vi "Frequency Changer.vi"() -> ()   [LabVIEW 2025]
uses:
  Globals/Speaker VISA Global.vi
  Globals/Motor VISA Global.vi
  Globals/Wire VISA Global.vi
  Globals/Light VISA Global.vi
  Globals/Solenoid VISA Global.vi
  Globals/Touch VISA Global.vi
panel:
  out "Success?":bool
  in  "Cancel Button":bool
  in  "OK Button":bool
  in  "Frequency":i16
  in  "Module":string(combo)
  # "Frequency is in bits per second, except solenoid, which is bytes per second"
  # "Max Frequencies:\nSound: TBD\nMotor: TBD\nWire: 800\nLight: 800\nSolenoid: 16\nTouch: 800"
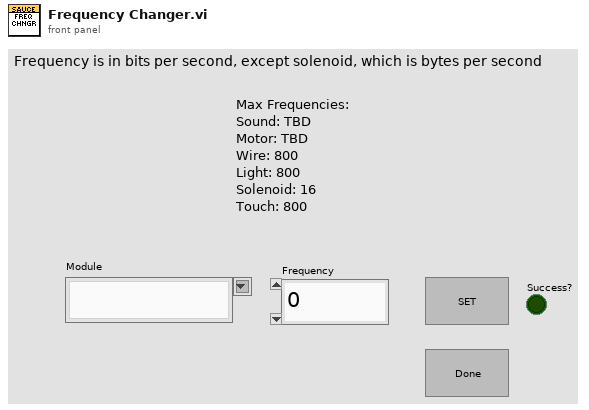
[diagram p1: front panel]
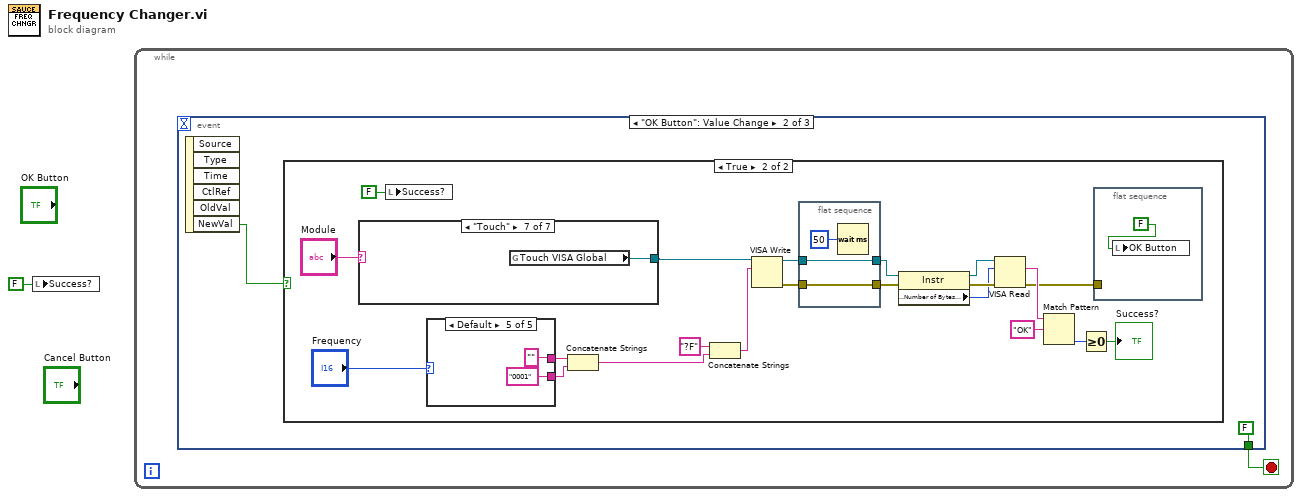
[diagram p0: block diagram]
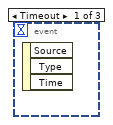
[diagram p2: hidden frame]
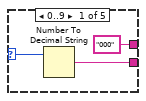
[diagram p4: hidden frame]
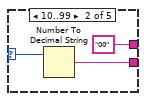
[diagram p5: hidden frame]
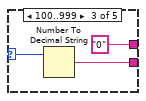
[diagram p6: hidden frame]
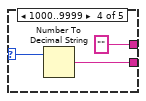
[diagram p7: hidden frame]
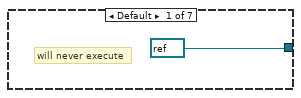
[diagram p8: hidden frame]
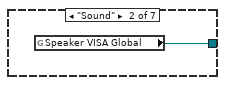
[diagram p9: hidden frame]
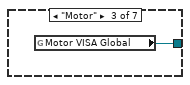
[diagram p10: hidden frame]
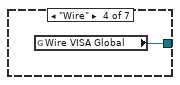
[diagram p11: hidden frame]
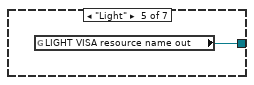
[diagram p12: hidden frame]
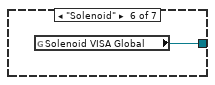
[diagram p13: hidden frame]
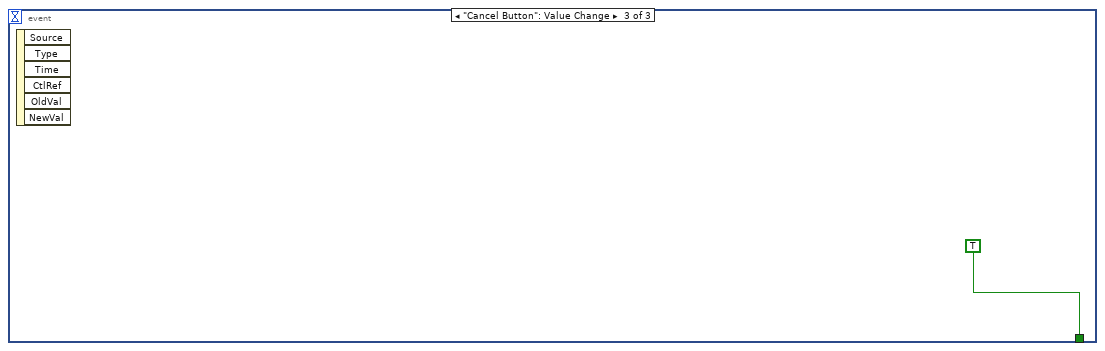
[diagram p14: hidden frame]
diagram:
  n1 = local write "Success?"(FALSE ("Success?")) -> ()
  n2 = while {
    stop <- w2 stop-if-true
    n3 = event shown="[1] \"OK Button\": Value Change" {
      selector: _ -> [_ _ _]
      dyn-events: _ -> [_ _ _]
      timeout: _ -> [_ _ _]
      tunnel: [_ FALSE TRUE] -> w2
      event Timeout {
        n4 = event-data() -> ()  [unwired: 1 in, 3 out]
      }
      event "OK Button": Value Change {
        n5 = event-data() -> ("NewVal"=w4:bool)  [unwired: 1 in, 5 out]
        n6 = case shown="True" w4 {
          frame False {
          }
          frame True {
            n7 = case shown="\"Touch\"" "Module" {
              tunnel: [refnum<visa-resource-name> refnum ("VISA resource name") w45 w46 w47 w48 w49 w50] -> w6
              frame Default {
                # "will never execute"
              }
              frame "Sound" {
                n8 = global read "Speaker VISA Global.vi" "Speaker VISA Global"() -> (w45:refnum<visa-resource-name>)
              }
              frame "Motor" {
                n9 = global read "Motor VISA Global.vi" "Motor VISA Global"() -> (w46:refnum<visa-resource-name>)
              }
              frame "Wire" {
                n10 = global read "Wire VISA Global.vi" "Wire VISA Global"() -> (w47:refnum<visa-resource-name>)
              }
              frame "Light" {
                n11 = global read "Light VISA Global.vi" "LIGHT VISA resource name out"() -> (w48:refnum<visa-resource-name>)
              }
              frame "Solenoid" {
                n12 = global read "Solenoid VISA Global.vi" "Solenoid VISA Global"() -> (w49:refnum<visa-resource-name>)
              }
              frame "Touch" {
                n13 = global read "Touch VISA Global.vi" "Touch VISA Global"() -> (w50:refnum<visa-resource-name>)
              }
            }
            n14 = local write "Success?"(FALSE ("Success?")) -> ()
            n15 = case shown="Default" "Frequency" {
              selector: "Frequency" -> [w29 w32 w35 w38 _]
              tunnel: [w28 w31 w34 w37 "0001"] -> w14
              tunnel: ["000" "00" "0" "" ""] -> w13
              frame 0..9 {
                n16 = Number To Decimal String(number=w29) -> (decimal integer string=w28:string)  [unwired: 1 in]
              }
              frame 10..99 {
                n17 = Number To Decimal String(number=w32) -> (decimal integer string=w31:string)  [unwired: 1 in]
              }
              frame 100..999 {
                n18 = Number To Decimal String(number=w35) -> (decimal integer string=w34:string)  [unwired: 1 in]
              }
              frame 1000..9999 {
                n19 = Number To Decimal String(number=w38) -> (decimal integer string=w37:string)  [unwired: 1 in]
              }
              frame Default {
              }
            }
            n20 = Concatenate Strings(w13, w14) -> (w12:string)
            n21 = Concatenate Strings("?F" ("string"), w12) -> (w17:string)
            n22 = VISA Write(VISA resource name=w6, write buffer=w17) -> (VISA resource name out=w23:refnum<visa-resource-name>, error out=w24:errorcluster)  [unwired: 1 in, 1 out]
            n23 = flat-sequence {
              tunnel: w24 -> [w42]
              tunnel: [w42] -> w22
              tunnel: [w41] -> w21
              tunnel: w23 -> [w41]
              frame #0 {
                n24 = Wait (ms)(milliseconds to wait=u32 50) -> ()  [unwired: 1 out]
              }
            }
            n25 = property class="Instr"(reference=w21, error in=w22) -> (reference out=w19:refnum<visa-resource-name>, error out=w20:errorcluster, "Serial Settings:Number of Bytes at Serial Port"=w18:u32)
            n26 = VISA Read(VISA resource name=w19, byte count=w18, error in (no error)=w20) -> (read buffer=w11:string, error out=w5:errorcluster)  [unwired: 2 out]
            n27 = Match Pattern(string=w11, regular expression="OK") -> (offset past match=w9:i32)  [unwired: 1 in, 3 out]
            n28 = Greater Or Equal To 0?(x=w9) -> (x >= 0?=→"Success?":bool)
            n29 = flat-sequence {
              tunnel: w5 -> [_]
              frame #0 {
                n30 = local write "OK Button"(FALSE) -> ()
              }
            }
          }
        }
      }
      event "Cancel Button": Value Change {
        n31 = event-data() -> ()  [unwired: 1 in, 6 out]
      }
    }
  }
